vi "Trim Data.vi"(0 "length":u32=20, 1 "Boolean":bool, 5 "Trim Data Ref":refnum<vi>, 11 "Pretrigger Size":i32, 12 "Array":sgl[][](array[numeric])) -> (3 "Data Out":sgl[][](array[numeric]), 13 "Current Size":dbl, 14 "Elements Deleted":dbl)   [LabVIEW 2019]
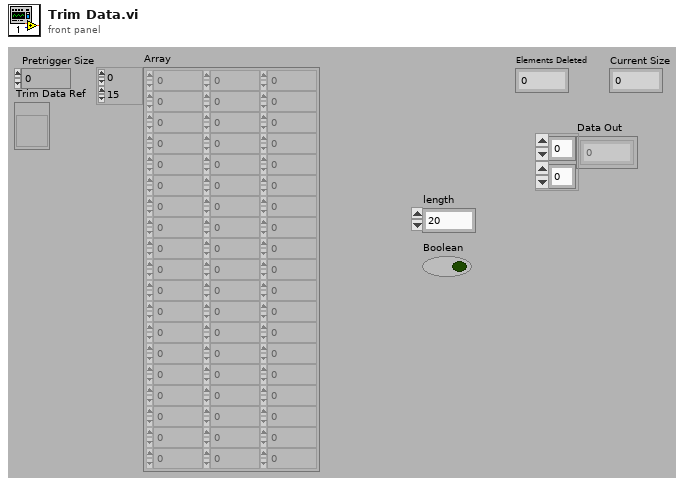
[diagram p1: front panel]
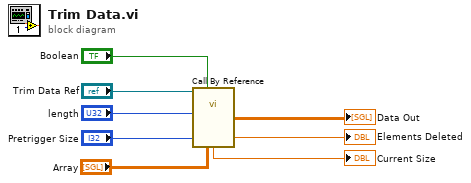
[diagram p0: block diagram]
diagram:
  n1 = call-by-ref "?"(reference="Trim Data Ref", "length"="length", "Boolean"="Boolean", "Pretrigger Size"="Pretrigger Size", "Array"="Array") -> ("Data Out"=→"Data Out":sgl[][], "Current Size"=→"Current Size":dbl, "Elements Deleted"=→"Elements Deleted":dbl)  [unwired: 10 in, 2 out]
